vi "Tosca-Initialize Accumulators.vi"(7 "Input Events":T1[](array[typedef])) -> (8 "Accumulators":T5[](array[typedef]))   [LabVIEW 2020]
uses:
  Typedefs/Tosca-Accumulator State.ctl
  Digital Input VIs/Tosca-Input Event.ctl
  Digital Input VIs/Tosca-Input Criterion.ctl
  epl-vi-lib/Utility VIs/Type Defs/Logic State.ctl
  Typedefs/Tosca-Accumulator.ctl
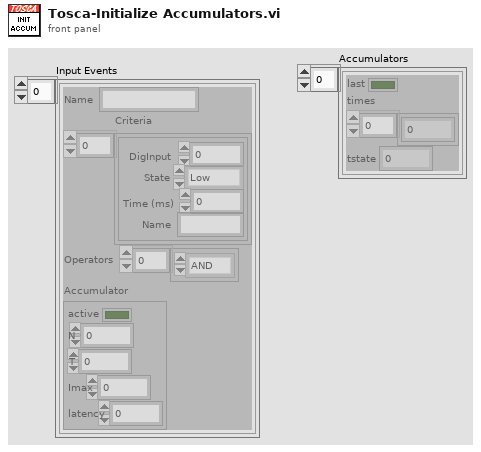
[diagram p1: front panel]
types:
  T1 = typedef "Tosca-Input Event.ctl" = cluster{"Name":string, "Criteria":T2[], "Operators":enum16{"AND", "OR"}[], "Accumulator":T4}
  T2 = typedef "Tosca-Input Criterion.ctl" = cluster{"DigInput":i32, "State":T3, "Time (ms)":i32, "Name":string}
  T3 = typedef "Logic State.ctl" = enum16{"Low", "High", "Rising", "Falling"}
  T4 = typedef "Tosca-Accumulator.ctl" = cluster{"active":bool, "N":i32, "T":dbl, "Imax":dbl, "latency":dbl}
  T5 = typedef "Tosca-Accumulator State.ctl" = cluster{"last":bool, "times":dbl[], "tstate":dbl}
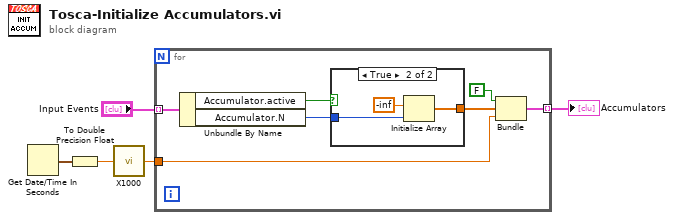
[diagram p0: block diagram]
diagram:
  n1 = Get Date/Time In Seconds() -> (seconds since 1Jan1904=w3:timestamp)
  n2 = To Double Precision Float(number=w3) -> (double precision float=w2:dbl)
  n3 = call "X1000.vi"("X"=w2) -> ("X/1000"=w1:dbl)
  n4 = for {
    tunnel: "Input Events" -> [w12] mode=indexing
    tunnel: [w7] -> w4 mode=indexing
    tunnel: w1 -> [w6]
    n5 = Unbundle By Name(w12) -> ("Accumulator.active"=w11:bool, "Accumulator.N"=w10:i32)
    n6 = case shown="True" w11 {
      tunnel: w10 -> [_ w15]
      tunnel: [_ w13] -> w9
      frame False {
      }
      frame True {
        n7 = Initialize Array(-inf, w15) -> (w13:dbl[])
      }
    }
    n8 = Bundle(FALSE, w9, "X/1000"=w6) -> (w7:cluster{bool, dbl[], "X/1000":dbl})  [unwired: 1 in]
  }
  "Accumulators" <- w4
